vi "flasher(SubVI).vi"(6 "Sample Rate":dbl, 9 "# Pulses":i32, 10 "Boolean":bool, 11 "Output channel (for flashing)":tag) -> ()   [LabVIEW 2013]
uses:
  <vilib>/DAQmx/write.llb/DAQmx Write (Analog 1D DBL 1Chan NSamp).vi
  <vilib>/DAQmx/create/channels.llb/DAQmx Create Channel (AO-Voltage-Basic).vi
  <vilib>/DAQmx/configure/timing.llb/DAQmx Timing (Sample Clock).vi
  <vilib>/DAQmx/miscellaneous.llb/DAQmx Fill In Error Info.vi
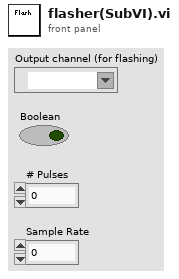
[diagram p1: front panel]
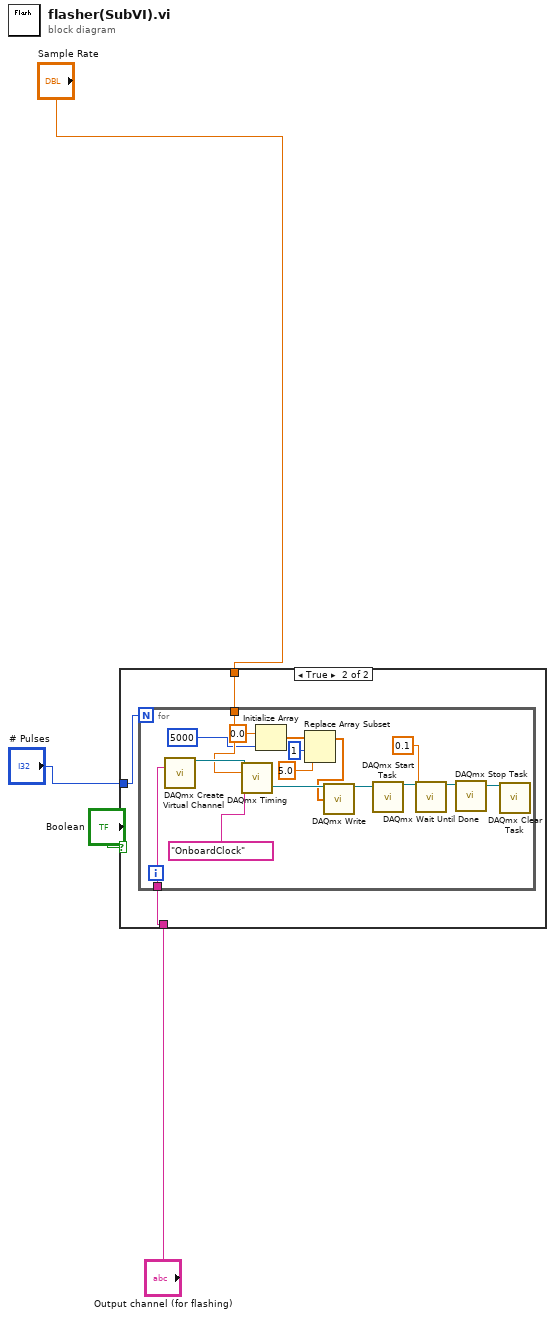
[diagram p0: block diagram]
diagram:
  n1 = case shown="True" "Boolean" {
    tunnel: "Output channel (for flashing)" -> [_ w7]
    tunnel: "Sample Rate" -> [_ w6]
    tunnel: "# Pulses" -> [_ w5]
    frame False {
    }
    frame True {
      n2 = for {
        N: w5 -> [_]
        tunnel: w7 -> [w23]
        tunnel: w6 -> [w20]
        n3 = call-poly <vilib>:"DAQmx Create Virtual Channel.vi"("physical channels"=w23) -> ("task out"=w21:refnum<k21>)  [unwired: 13 in, 1 out]
        n4 = call-poly <vilib>:"DAQmx Timing.vi"("task/channels in"=w21, "rate"=w20, "source"=tag "OnboardClock") -> ("task out"=w14:refnum<k21>)  [unwired: 11 in, 1 out]
        n5 = Initialize Array(0.0 ("element"), 5000 ("dimension size")) -> (w17:dbl[])
        n6 = Replace Array Subset(array=w17, new element=5.0 ("new element/subarray"), index=1) -> (w13:dbl[])
        n7 = call-poly <vilib>:"DAQmx Write.vi"("task/channels in"=w14, "data"=w13) -> ("task out"=w12:refnum<k21>)  [unwired: 11 in, 2 out]
        n8 = call <vilib>:"DAQmx Start Task.vi"("task/channels in"=w12) -> ("task out"=w11:refnum<k21>)  [unwired: 13 in, 1 out]
        n9 = call <vilib>:"DAQmx Wait Until Done.vi"("task/channels in"=w11, "timeout (sec)"=0.1) -> ("task out"=w10:refnum<k21>)  [unwired: 12 in, 1 out]
        n10 = call <vilib>:"DAQmx Stop Task.vi"("task/channels in"=w10) -> ("task out"=w22:refnum<k21>)  [unwired: 13 in, 1 out]
        n11 = call <vilib>:"DAQmx Clear Task.vi"("task in"=w22) -> ()  [unwired: 14 in, 1 out]
      }
    }
  }
